vi "Real LU Inverse Matrix.vi"(0 "LU Info":cluster{"LU":dbl[][], "Pivot":i32[]} {"LU" format="%.3f"}) -> (1 "Inverse Matrix":T1, 2 "error":i32)   [LabVIEW 2014, in "NI_AALBase.lvlib"]
doc: "Finds the inverse matix of the input matrix if it exists. If the input matrix is nonsingular, then the inverse matirx can be found by solving the linear system\n\n A B = I\n\n where\n A is the Input Matrix\n B is the Inverse Matrix\n I is the identity matirx."
uses:
  NI_AALBase.lvlib
  RealMatrix.ctl
  lvanlys.dll
  NI_Matrix.lvlib
panel:
  # "Real LU Inverse Matrix"
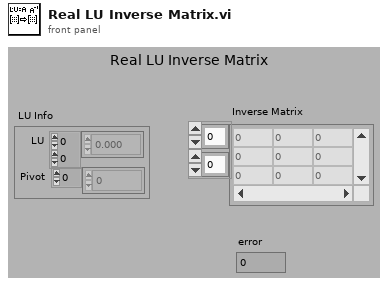
[diagram p1: front panel]
types:
  T1 = typedef "NI_Matrix.lvlib/RealMatrix.ctl" = dbl[][]
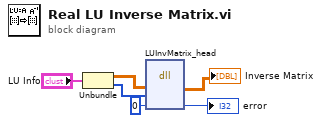
[diagram p0: block diagram]
diagram:
  n1 = Unbundle("LU Info") -> ("LU"=w4:dbl[][], "Pivot"=w3:i32[])
  n2 = dll-call lib="C:/Program Files (x86)/National Instruments/LabVIEW 2014/resource/lvanlys.*" fn="LUInvMatrix_head"("LU"=w4, "Pivot"=w3, "error"=0) -> ("LU"=→"Inverse Matrix":dbl[][], "error"=→"error":i32)  [unwired: 5 in, 2 out]
